vi "FisherPaykel Start Agitate Profile.vi"(0 "VISA Refnum in":refnum<visa-resource-name>, 1 "Agitate Parameters":T2 {"PauseTime (0-1800ms 10ms Increment)" step=10; "PlateauTime (0-1800ms 10ms Increment)" step=10; "TargetSpeed (0-200RPM)" max=1600 step=1; "RampUpTime (1-600ms)" max=600 step=10; "Agitate Running Time (sec)" step=1}, 2 "GEA2 Reference In":refnum<k24>, 5 "Error In":errorcluster, 7 "Main Command":T4=">GA", 8 "Debug":bool, 10 "Use GEA Inverter Output":bool, 13 "GEA Inputs":T1={"Source"=228, "Destination"=35} {"Destination" format="%.0x"; "Source" format="%.0x"}) -> (14 "VISA resource name out":refnum<visa-resource-name>, 16 "GEA2 Reference Out":refnum<k24>, 19 "Error Out":errorcluster)   [LabVIEW 2016]
uses:
  Type Definitions/Fisher Paykel Main Command.ctl
  Type Definitions/Fisher Paykel Agitate Parameters.ctl
  Type Definitions/FisherPaykel Direction CMD.ctl
  Trunk/Utility/LabVIEW GEA2 Toolkit v1.0.0.0/type defs/Source_Destination.ctl
  C:/Technology Lab/NI-2010/Trunk/Utility/LabVIEW GEA2 Toolkit v1.0.0.0/Appliance.NET/GeaCommunication.dll
  Trunk/Utility/LabVIEW GEA2 Toolkit v1.0.0.0/Appliance.NET/GeaCommunication.dll
  Trunk/Utility/LabVIEW GEA2 Toolkit v1.0.0.0/type defs/ERD Write Data In.ctl
  Trunk/Utility/LabVIEW GEA2 Toolkit v1.0.0.0/type defs/Data Type.ctl
  Trunk/Utility/LabVIEW GEA2 Toolkit v1.0.0.0/library/GEA2_Toolkit.lvlib
panel:
  out "Command (Debug)":string
  # "Agitate Profile Parameters"
  # "Agitate Start Parameters"
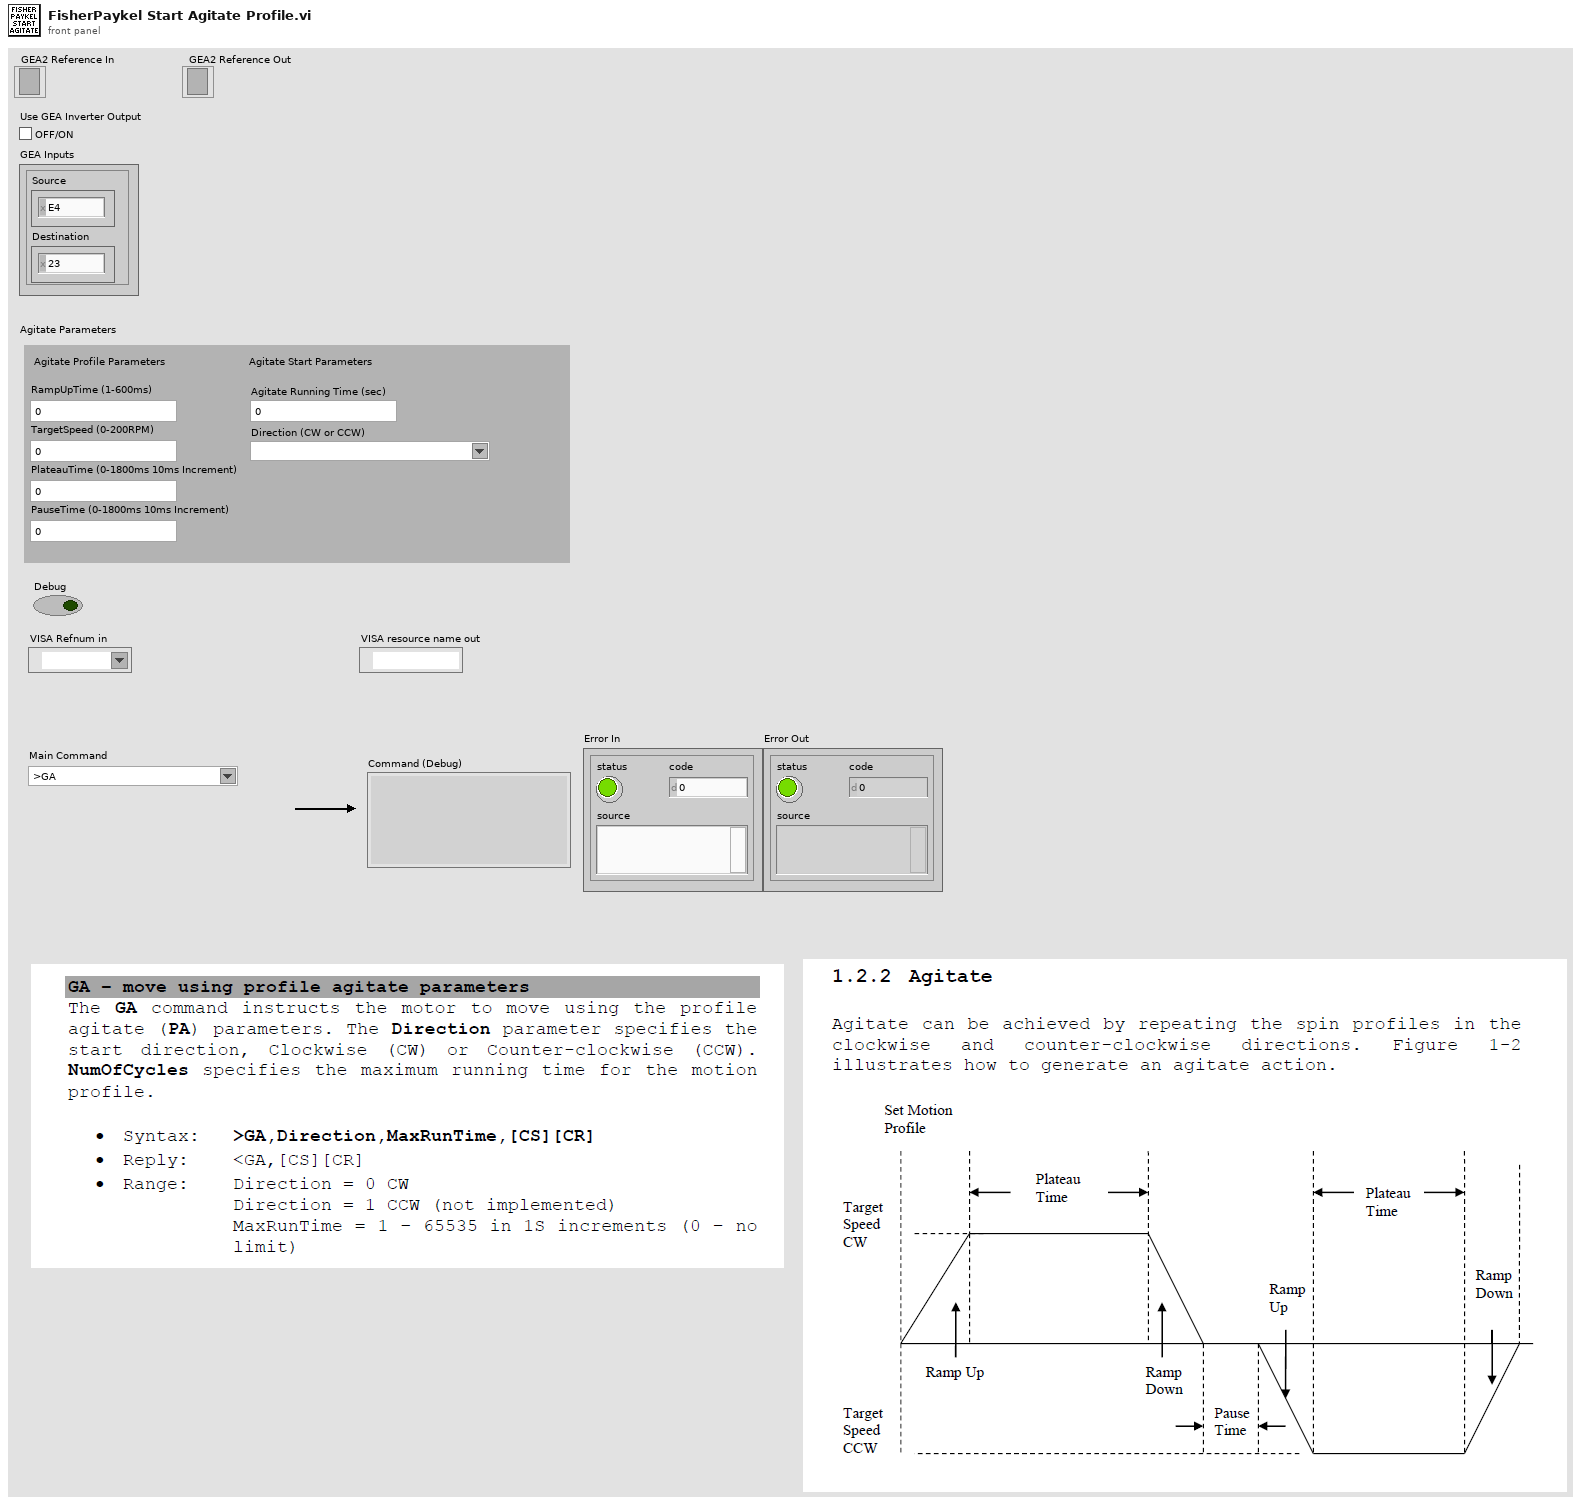
[diagram p1: front panel]
types:
  T1 = typedef "GEA2_Toolkit.lvlib/Source_Destination.ctl" = cluster{"Source":u8, "Destination":u8}
  T2 = typedef "Fisher Paykel Agitate Parameters.ctl" = cluster{"Agitate Running Time (sec)":u16, "Direction (CW or CCW)":T3, "RampUpTime (1-600ms)":u16, "TargetSpeed (0-200RPM)":u16, "PlateauTime (0-1800ms 10ms Increment)":u16, "PauseTime (0-1800ms 10ms Increment)":u16}
  T3 = typedef "FisherPaykel Direction CMD.ctl" = string
  T4 = typedef "Fisher Paykel Main Command.ctl" = string
  T5 = typedef "GEA2_Toolkit.lvlib/ERD Write Data In.ctl" = cluster{"ERD Number":u16, "Data Type":T6, "Data":string}
  T6 = typedef "GEA2_Toolkit.lvlib/Data Type.ctl" = enum16{"string", "boolean", "uint8_t", "uint16_t", "uint32_t", "uint64_t"}
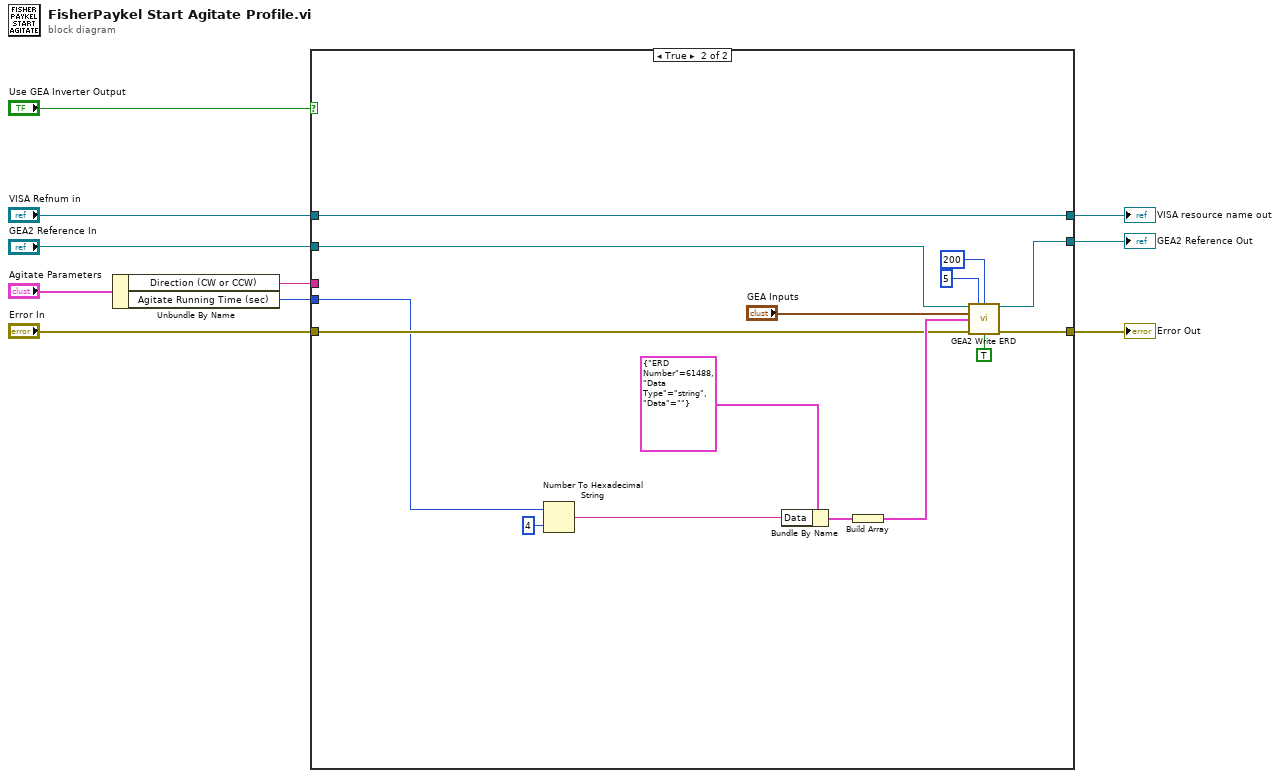
[diagram p0: block diagram]
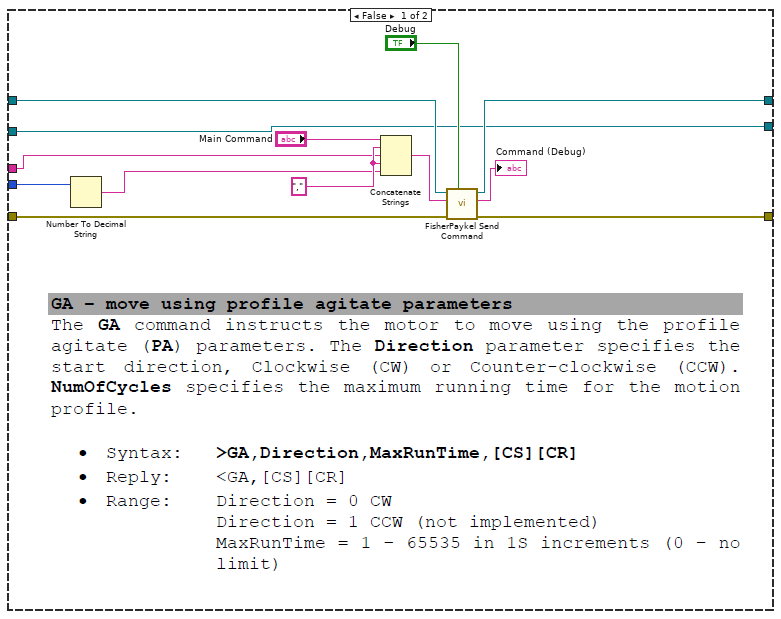
[diagram p2: hidden frame]
diagram:
  n1 = Unbundle By Name("Agitate Parameters") -> ("Direction (CW or CCW)"=w4:T3, "Agitate Running Time (sec)"=w5:u16)
  n2 = case shown="True" "Use GEA Inverter Output" {
    tunnel: [w23 w30] -> w10
    tunnel: "VISA Refnum in" -> [w22 w30]
    tunnel: "Error In" -> [w18 w29]
    tunnel: [w17 w28] -> w7
    tunnel: w5 -> [w15 w27]
    tunnel: w4 -> [w13 _]
    tunnel: "GEA2 Reference In" -> [w11 w26]
    tunnel: [w11 w25] -> w1
    frame False {
      w20 = ","
      n3 = Number To Decimal String(number=w15) -> (decimal integer string=w14:string)  [unwired: 1 in]
      n4 = Concatenate Strings("Main Command", w20, w13, w20, w14) -> (w19:string)
      n5 = call "FisherPaykel Send Command.vi"("Debug"="Debug", "error in (no error)"=w18, "Send Command"=w19, "VISA Refnum in"=w22) -> ("error out"=w17:errorcluster, "Command (Debug)"=→"Command (Debug)":string, "VISA Refnum out"=w23:refnum<visa-resource-name>)  [unwired: 5 in]
    }
    frame True {
      n6 = Number To Hexadecimal String(1:i16 4 ("width (-)"), 2:w27) -> (0:w24:string)
      n7 = Bundle By Name(cluster=T5 {"ERD Number"=61488, "Data Type"=enum."string", "Data"=""} ("ERD Write Data In"), "Data"=w24) -> (w32:T5)
      n8 = Build Array(w32) -> (w34:T5[])
      n9 = call "GEA2 Write ERD.vi"("GEA2 Reference In"=w26, "Retry Count"=5, "Read Timeout (ms)"=u32 200, "GEA Inputs"="GEA Inputs", "Write ERD List"=w34, "Error In"=w29, "Verify ERD Response?"=TRUE) -> ("GEA2 Reference Out"=w25:refnum<k24>, "Error Out"=w28:errorcluster)  [unwired: 6 in, 1 out]
    }
  }
  "Error Out" <- w7
  "VISA resource name out" <- w10
  "GEA2 Reference Out" <- w1
